vi "ProFile_guided_Ablation_Burst_FindFocus.vi"(1 "z-step":sgl=1.75, 2 "Error In":errorcluster, 3 "z-offset":sgl=1.75) -> (0 "error out":errorcluster caption="error Out")   [LabVIEW 2016]
doc: "2D motor scan example Vi."
uses:
  Utility/Global Constants.vi
  <vilib>/Utility/file.llb/Read From Spreadsheet File (DBL).vi
  Utility/Global_Stage.vi
panel:
  out "RS":bool
  out "Read out":sgl[][](array[numeric])
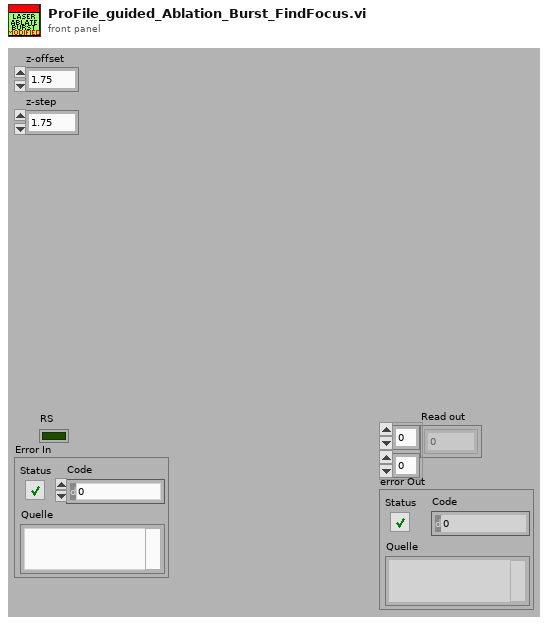
[diagram p1: front panel]
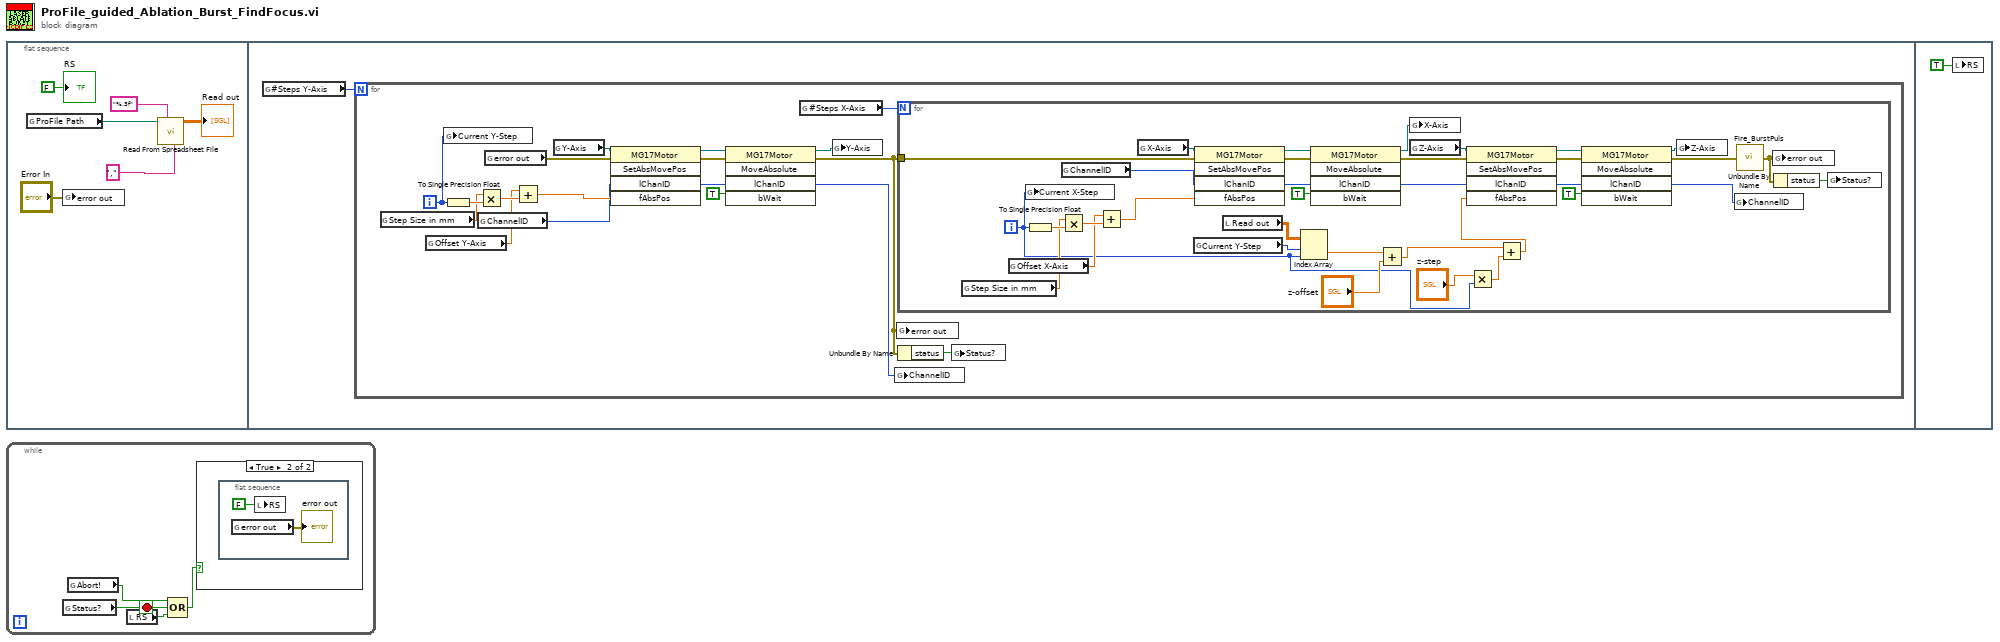
[diagram p0: block diagram]
diagram:
  n1 = flat-sequence {
    frame #0 {
      n2 = global read "Global Constants.vi" "ProFile Path"() -> (w6:path)
      n3 = global write "Global Constants.vi" "error out"("Error In") -> ()
      n4 = call-poly <vilib>:"Read From Spreadsheet File.vi"("delimiter (\\t)"="," ("delimiter (\\t)"), "format (%.3f)"="%.3f", "file path (dialog if empty)"=w6) -> ("all rows"=→"Read out":dbl[][])  [unwired: 4 in, 4 out]
      "RS" <- FALSE
    }
    frame #1 {
      n5 = global read "Global Constants.vi" "#Steps Y-Axis"() -> (w7:i32)
      n6 = for {
        N: w7 -> [_]
        i -> [w10]
        n7 = global read "Global Constants.vi" "Step Size in mm"() -> (w12:sgl)
        n8 = global read "Global Constants.vi" "Offset Y-Axis"() -> (w13:sgl)
        n9 = global write "Global Constants.vi" "Current Y-Step"(w10) -> ()
        n10 = To Single Precision Float(number=w10) -> (single precision float=w22:sgl)
        n11 = Multiply(x=w12, y=w22) -> (x*y=w20:sgl)
        n12 = global read "Global_Stage.vi" "ChannelID"() -> (w16:i32)
        n13 = global read "Global Constants.vi" "error out"() -> (w8:errorcluster)
        n14 = Add(x=w13, y=w20) -> (x+y=w19:sgl)
        n15 = global read "Global_Stage.vi" "Y-Axis"() -> (w18:refnum<k7>)
        n16 = invoke class="MG17Motor" method="SetAbsMovePos"(reference=w18, error in=w8, "lChanID"=w16, "fAbsPos"=w19) -> (reference out=w21:refnum<k7>, error out=w25:errorcluster, "lChanID"=w23:i32)  [unwired: 1 in, 2 out]
        n17 = invoke class="MG17Motor" method="MoveAbsolute"(reference=w21, error in=w25, "lChanID"=w23, "bWait"=TRUE) -> (reference out=w17:refnum<k7>, error out=w9:errorcluster, "lChanID"=w14:i32)  [unwired: 1 in, 2 out]
        n18 = global read "Global Constants.vi" "#Steps X-Axis"() -> (w11:i32)
        n19 = global write "Global_Stage.vi" "Y-Axis"(w17) -> ()
        n20 = global write "Global_Stage.vi" "ChannelID"(w14) -> ()
        n21 = global write "Global Constants.vi" "error out"(w9) -> ()
        n22 = for {
          N: w11 -> [_]
          tunnel: w9 -> [w33]
          i -> [w28]
          n23 = global read "Global Constants.vi" "Step Size in mm"() -> (w37:sgl)
          n24 = global read "Global Constants.vi" "Offset X-Axis"() -> (w36:sgl)
          n25 = global write "Global Constants.vi" "Current X-Step"(w28) -> ()
          n26 = To Single Precision Float(number=w28) -> (single precision float=w56:sgl)
          n27 = Multiply(x=w37, y=w56) -> (x*y=w48:sgl)
          n28 = global read "Global_Stage.vi" "ChannelID"() -> (w42:i32)
          n29 = Add(x=w36, y=w48) -> (x+y=w47:sgl)
          n30 = global read "Global_Stage.vi" "X-Axis"() -> (w43:refnum<k7>)
          n31 = global read "Global Constants.vi" "Current Y-Step"() -> (w34:i32)
          n32 = invoke class="MG17Motor" method="SetAbsMovePos"(reference=w43, error in=w33, "lChanID"=w42, "fAbsPos"=w47) -> (reference out=w51:refnum<k7>, error out=w59:errorcluster, "lChanID"=w58:i32)  [unwired: 1 in, 2 out]
          n33 = local read "Read out"() -> (w35:sgl[][])
          n34 = Index Array(array=w35, index (row)=w34, index (col)=w28) -> (element=w32:sgl)
          n35 = invoke class="MG17Motor" method="MoveAbsolute"(reference=w51, error in=w59, "lChanID"=w58, "bWait"=TRUE) -> (reference out=w40:refnum<k7>, error out=w52:errorcluster, "lChanID"=w50:i32)  [unwired: 1 in, 2 out]
          n36 = Add(x=w32, y="z-offset") -> (x+y=w30:sgl)
          n37 = global write "Global_Stage.vi" "X-Axis"(w40) -> ()
          n38 = global read "Global_Stage.vi" "Z-Axis"() -> (w41:refnum<k7>)
          n39 = Multiply(x="z-step", y=w28) -> (x*y=w27:sgl)
          n40 = Add(x=w30, y=w27) -> (x+y=w26:sgl)
          n41 = invoke class="MG17Motor" method="SetAbsMovePos"(reference=w41, error in=w52, "lChanID"=w50, "fAbsPos"=w26) -> (reference out=w49:refnum<k7>, error out=w55:errorcluster, "lChanID"=w53:i32)  [unwired: 1 in, 2 out]
          n42 = invoke class="MG17Motor" method="MoveAbsolute"(reference=w49, error in=w55, "lChanID"=w53, "bWait"=TRUE) -> (reference out=w39:refnum<k7>, error out=w46:errorcluster, "lChanID"=w38:i32)  [unwired: 1 in, 2 out]
          n43 = global write "Global_Stage.vi" "Z-Axis"(w39) -> ()
          n44 = global write "Global_Stage.vi" "ChannelID"(w38) -> ()
          n45 = call "Fire_BurstPuls.vi"("error in"=w46) -> ("error out"=w44:errorcluster)
          n46 = global write "Global Constants.vi" "error out"(w44) -> ()
          n47 = Unbundle By Name(w44) -> ("status"=w45:bool)
          n48 = global write "Global Constants.vi" "Status?"(w45) -> ()
        }
        n49 = Unbundle By Name(w9) -> ("status"=w15:bool)
        n50 = global write "Global Constants.vi" "Status?"(w15) -> ()
      }
    }
    frame #2 {
      n51 = local write "RS"(TRUE) -> ()
    }
  }
  n52 = while {
    stop <- w61 stop-if-true
    n53 = global read "Global Constants.vi" "Status?"() -> (w63:bool)
    n54 = global read "Global Constants.vi" "Abort!"() -> (w64:bool)
    n55 = local read "RS"() -> (w62:bool)
    n56 = Compound Arithmetic op=OR(w64, w63, w62) -> (w61:bool)
    n57 = case shown="True" w61 {
      frame False {
      }
      frame True {
        n58 = flat-sequence {
          frame #0 {
            n59 = global read "Global Constants.vi" "error out"() -> (→"error out":errorcluster)
            n60 = local write "RS"(FALSE) -> ()
          }
        }
      }
    }
  }
